vi "Config Display.vi"(0 "VISA resource name":refnum<visa-resource-name>, 5 "Display Field (1)":dbl=1.0 min=1.0 max=8.0 step=1.0, 7 "Input to Display(1:1)":u16(ring)=1 items=["None", "1", "2", "3", "4", "5", "6", "7", "8"], 9 "Source (0:Kelvin)":u16(ring) items=["Kelvin", "Celsius", "Sensor Units", "Linear Data", "Min Data", "Max Data"], 11 "error in (no error)":errorcluster) -> (4 "VISA resource name out":refnum<visa-resource-name>, 15 "error out":errorcluster)   [LabVIEW 2017, in "Lake Shore Cryotronics 218.lvlib"]
doc: "This VI configures Display Field parameters."
uses:
  Lake Shore Cryotronics 218.lvlib
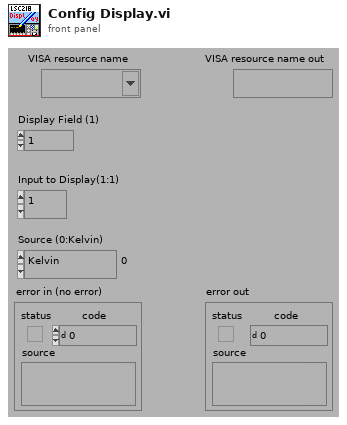
[diagram p1: front panel]
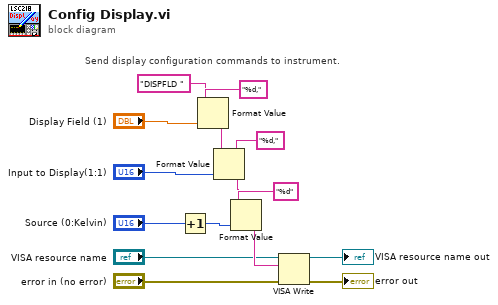
[diagram p0: block diagram]
diagram:
  # "Send display configuration commands to instrument."
  n1 = Increment(x="Source (0:Kelvin)") -> (x+1=w5:u16)
  n2 = Format Value(string ("")="DISPFLD ", format string="%d,", value (0)="Display Field (1)") -> (output string=w8:string)
  n3 = Format Value(string ("")=w8, format string="%d,", value (0)="Input to Display(1:1)") -> (output string=w7:string)
  n4 = Format Value(string ("")=w7, format string="%d", value (0)=w5) -> (output string=w6:string)
  n5 = VISA Write(VISA resource name="VISA resource name", write buffer=w6, error in (no error)="error in (no error)") -> (VISA resource name out=→"VISA resource name out":refnum<visa-resource-name>, error out=→"error out":errorcluster)  [unwired: 1 out]
